vi "DriveGlobal.vi"() -> ()   [LabVIEW 2020]
doc: "Global variables for drive"
panel:
  out "RightMotorOutput":dbl
  out "LeftMotorOutput":dbl
  in  "RSpeed Demand (ft/s)":dbl
  in  "LSpeed Demand (ft/s)":dbl
  in  "Gyro Z":dbl
  in  "Gyro Y":dbl
  in  "Gyro X":dbl
  in  "Right dist (ft)":dbl
  in  "Left dist (ft)":dbl
  in  "Right speed (ft/s)":dbl
  in  "Left speed (ft/s)":dbl
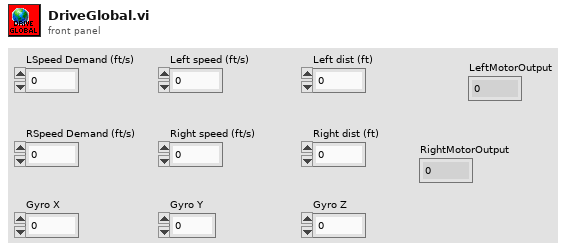
[diagram p1: front panel]
diagram:
